vi "Untitled 2.vi"() -> ()   [LabVIEW 2019]
panel:
  out "sin(x)":dbl
  in  "x":dbl
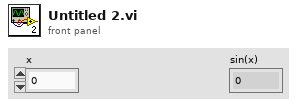
[diagram p1: front panel]
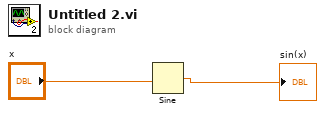
[diagram p0: block diagram]
diagram:
  n1 = Sine(x="x") -> (sin(x)=→"sin(x)":dbl)
